vi "SDG60ConfArbWaveform2new.vi"(0 "VISA resource name":refnum<visa-resource-name>="USB0::0xF4EC::0x1101::SDG6XEBC5R0119::INSTR", 1 "DDS/TArb 0: DDS":i32(ring) items=["DDS", "TrueArb"], 2 "Interpolation 0: Zero-order":i32(ring) items=["Zero-Order", "Linear", "Sinc", "Sin27", "Sinc13"], 3 "Offset (0.00 V)":dbl min=-10.0 max=10.0 format="%#_15g", 5 "Select Channel (1:Channel 1)":i32(ring)=1 items=["Channel 1"=1, "Channel 2"=2], 7 "Amplitude(0.1 Vpp)":dbl=0.1 min=0.001 max=20.0 step=1.0 format="%#.15f", 9 "Freq/SR/P (1 Hz)":dbl=1.0 min=1e-06 max=160000000.0 step=1.0 format="%#.15g", 11 "error in (no error)":errorcluster, 12 "Select Freq/SR/P (0:Freq)":i32(ring) items=["Frequency", "Sample Rate", "Period"], 13 "Phase (0 deg)":dbl min=-360.0 max=360.0 format="%#.15g") -> (4 "VISA resource name out":refnum<visa-resource-name>, 15 "error out":errorcluster)   [LabVIEW 2018]
doc: "Sets the waveform parameters for an arbitrary waveform. This VI should be called after <b>Create Arbitrary Waveform.vi</b> (for user defined arbitrary waveform) and <b>Select Arbitrary Waveform.vi</b>"
panel:
  # "Must precede with SDG60SelectArbitraryWFM\nMay take time (~20s) if WFM is large"
  # "Sinc type interpolations use virtual keys\nVirtual keys not used for zero-hold & linear\nInterpolation method, is only for TrueArb\nIf still selected, generator will not make any parameter changes"
  # "Range: 2mVpp-20Vpp. \n6 digits precision"
  # "Range: -10V-10V\n6 digits precision"
  # "Freq (DDS): 1uHz-50MHz \nFreq (TrueArb): 1uHz- Max depends on WFM length\nSR: 1uS/s-300MSa/s\nP: 20ns-1Ms\n10 Digit precision for F & SR\n6 Digit precision for P"
  # "For TrueArb use only F or SR \nFor DDS use F or P\nMay take time (few seconds!) to switch to TrueArb if WFM is large"
  # "Range -360..360deg, larger values will be warped to this range. Resolution 0.0001 deg"
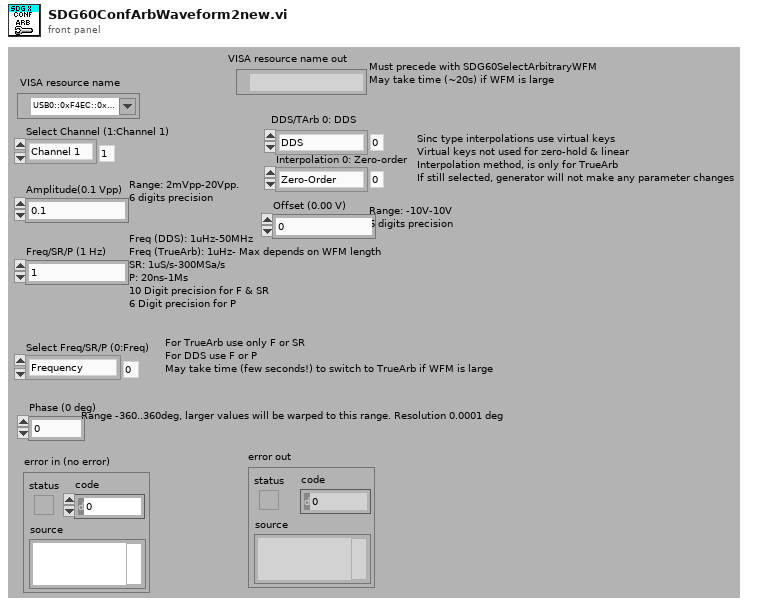
[diagram p1: front panel]
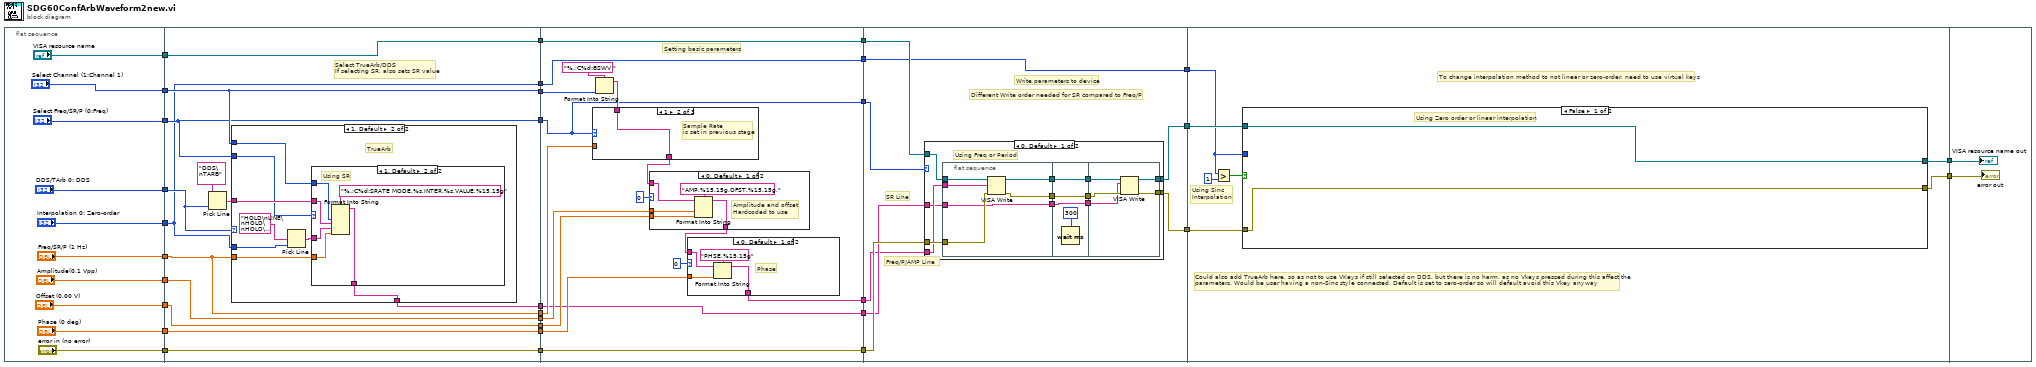
[diagram p0: block diagram]
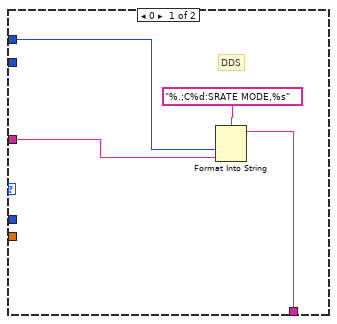
[diagram p2: hidden frame]
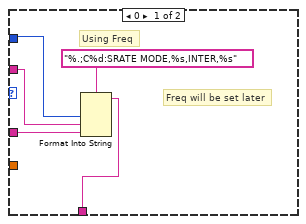
[diagram p3: hidden frame]
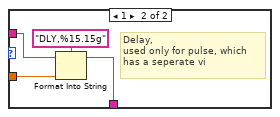
[diagram p4: hidden frame]
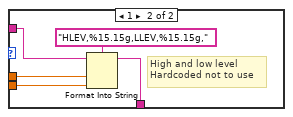
[diagram p5: hidden frame]
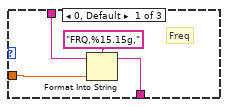
[diagram p6: hidden frame]
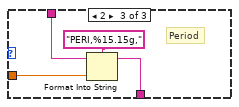
[diagram p7: hidden frame]
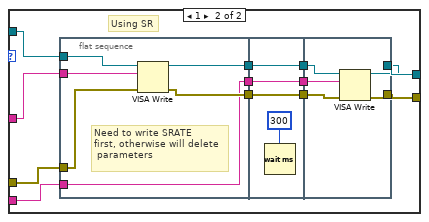
[diagram p8: hidden frame]
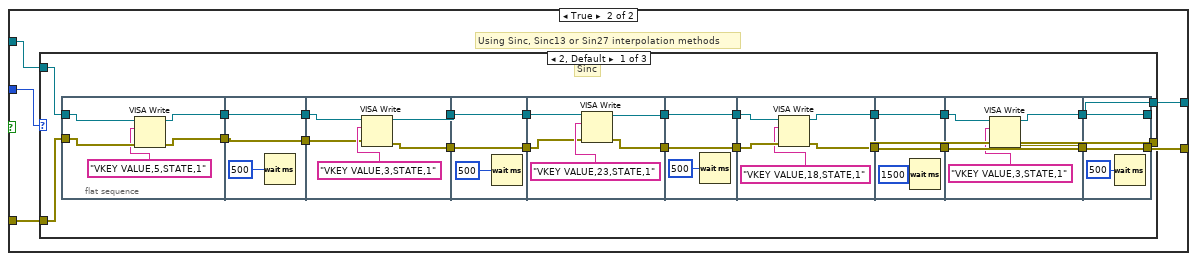
[diagram p9: hidden frame]
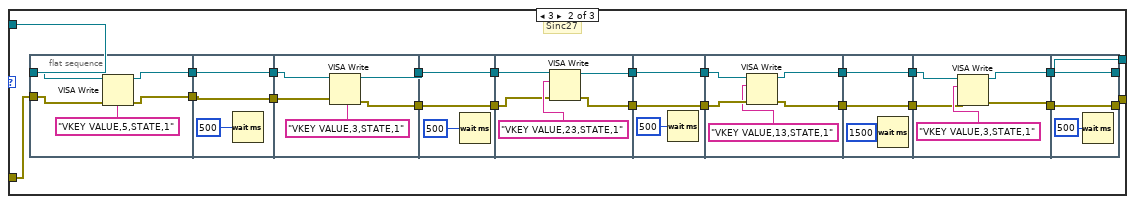
[diagram p10: hidden frame]
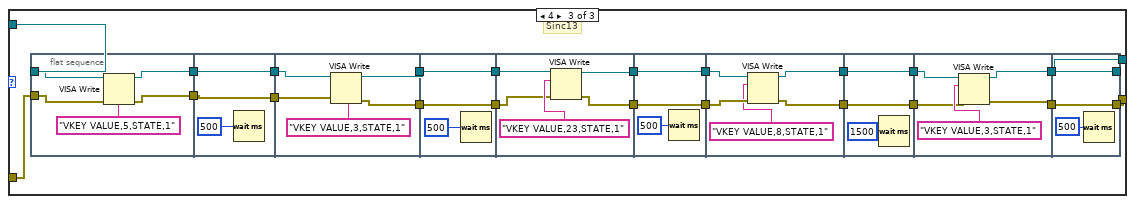
[diagram p11: hidden frame]
diagram:
  n1 = flat-sequence {
    tunnel: ["VISA resource name"] -> w31
    tunnel: ["error in (no error)"] -> w30
    tunnel: ["Amplitude(0.1 Vpp)"] -> w29
    tunnel: ["Phase (0 deg)"] -> w28
    tunnel: ["Freq/SR/P (1 Hz)"] -> w27
    tunnel: ["Offset (0.00 V)"] -> w26
    tunnel: ["Select Freq/SR/P (0:Freq)"] -> w25
    tunnel: ["DDS/TArb 0: DDS"] -> w24
    tunnel: ["Interpolation 0: Zero-order"] -> w23
    tunnel: ["Select Channel (1:Channel 1)"] -> w22
    tunnel: w31 -> [w50]
    tunnel: w30 -> [w54]
    tunnel: w29 -> [w48]
    tunnel: w28 -> [w49]
    tunnel: w27 -> [w47]
    tunnel: w26 -> [w46]
    tunnel: w25 -> [w44]
    tunnel: w24 -> [w51]
    tunnel: w23 -> [w43]
    tunnel: w22 -> [w45]
    tunnel: [w54] -> w21
    tunnel: [w50] -> w19
    tunnel: [w49] -> w17
    tunnel: [w48] -> w16
    tunnel: [w47] -> w15
    tunnel: [w46] -> w14
    tunnel: [w45] -> w13
    tunnel: [w44] -> w12
    tunnel: [w43] -> w11
    tunnel: [w42] -> w9
    tunnel: w21 -> [w94]
    tunnel: [w94] -> w20
    tunnel: w19 -> [w93]
    tunnel: [w93] -> w18
    tunnel: w17 -> [w84]
    tunnel: w16 -> [w86]
    tunnel: w15 -> [w87]
    tunnel: w14 -> [w85]
    tunnel: w13 -> [w88]
    tunnel: w12 -> [w78]
    tunnel: w11 -> [w83]
    tunnel: [w83] -> w10
    tunnel: w9 -> [w82]
    tunnel: [w82] -> w8
    tunnel: [w81] -> w7
    tunnel: [w78] -> w1
    tunnel: w20 -> [w129]
    tunnel: w18 -> [w126]
    tunnel: w10 -> [w123]
    tunnel: w8 -> [w125]
    tunnel: w7 -> [w124]
    tunnel: [w128] -> w6
    tunnel: [w127] -> w5
    tunnel: [w123] -> w4
    tunnel: w1 -> [w122]
    tunnel: w6 -> [w188]
    tunnel: w5 -> [w189]
    tunnel: w4 -> [w184]
    tunnel: [w190] -> w3
    tunnel: [w187] -> w2
    tunnel: w3 -> [w385]
    tunnel: w2 -> [w384]
    frame #0 {
    }
    frame #1 {
      # "Select TrueArb/DDS\nIf selecting SR, also sets SR value"
      n2 = Pick Line(multi-line string="DDS\nTARB", line index=w51) -> (output string=w52:string)  [unwired: 1 in]
      n3 = case shown="1, Default" w51 {
        tunnel: [w57 w66] -> w42
        tunnel: w45 -> [w55 w65]
        tunnel: w52 -> [w56 w64]
        tunnel: w47 -> [_ w61]
        tunnel: w44 -> [_ w60]
        tunnel: w43 -> [_ w59]
        frame 0 {
          # "DDS"
          n4 = Format Into String(format string="%.;C%d:SRATE MODE,%s", w55, w56) -> (resulting string=w57:string)  [unwired: 2 in, 1 out]
        }
        frame 1, Default {
          # "TrueArb"
          n5 = Pick Line(multi-line string="HOLD\nLINE\nHOLD\nHOLD\nHOLD\nHOLD", line index=w59) -> (output string=w62:string)  [unwired: 1 in]
          n6 = case shown="1, Default" w60 {
            tunnel: w65 -> [w70 w76]
            tunnel: [w69 w75] -> w66
            tunnel: w64 -> [w68 w74]
            tunnel: w62 -> [w67 w73]
            tunnel: w61 -> [_ w72]
            frame 0 {
              # "Freq will be set later"
              # "Using Freq"
              n7 = Format Into String(format string="%.;C%d:SRATE MODE,%s,INTER,%s", w70, w68, w67) -> (resulting string=w69:string)  [unwired: 2 in, 1 out]
            }
            frame 1, Default {
              # "Using SR"
              n8 = Format Into String(format string="%.;C%d:SRATE MODE,%s,INTER,%s,VALUE,%15.15g", w76, w74, w73, w72) -> (resulting string=w75:string)  [unwired: 2 in, 1 out]
            }
          }
        }
      }
    }
    frame #2 {
      # "Setting basic parameters"
      n9 = Format Into String(format string="%.;C%d:BSWV ", w88) -> (resulting string=w90:string)  [unwired: 2 in, 1 out]
      n10 = case shown="1" w78 {
        tunnel: w90 -> [w116 w117 w121]
        tunnel: [w114 w117 w119] -> w79
        tunnel: w87 -> [w113 _ w118]
        frame 0, Default {
          # "Freq"
          n11 = Format Into String(format string="FRQ,%15.15g,", initial string=w116, w113) -> (resulting string=w114:string)  [unwired: 1 in, 1 out]
        }
        frame 1 {
          # "Sample Rate\nis set in previous stage"
        }
        frame 2 {
          # "Period"
          n12 = Format Into String(format string="PERI,%15.15g,", initial string=w121, w118) -> (resulting string=w119:string)  [unwired: 1 in, 1 out]
        }
      }
      n13 = case shown="0, Default" 0 {
        tunnel: [w106 w111] -> w80
        tunnel: w86 -> [w105 w110]
        tunnel: w85 -> [w104 w109]
        tunnel: w79 -> [w103 w108]
        frame 0, Default {
          # "Amplitude and offset\nHardcoded to use"
          n14 = Format Into String(format string="AMP,%15.15g,OFST,%15.15g,", initial string=w103, w105, w104) -> (resulting string=w106:string)  [unwired: 1 in, 1 out]
        }
        frame 1 {
          # "High and low level\nHardcoded not to use"
          n15 = Format Into String(format string="HLEV,%15.15g,LLEV,%15.15g,", initial string=w108, w110, w109) -> (resulting string=w111:string)  [unwired: 1 in, 1 out]
        }
      }
      n16 = case shown="0, Default" 0 {
        tunnel: [w97 w101] -> w81
        tunnel: w84 -> [w96 w100]
        tunnel: w80 -> [w95 w99]
        frame 0, Default {
          # "Phase"
          n17 = Format Into String(format string="PHSE,%15.15g", initial string=w95, w96) -> (resulting string=w97:string)  [unwired: 1 in, 1 out]
        }
        frame 1 {
          # "Delay,\nused only for pulse, which \nhas a seperate vi"
          n18 = Format Into String(format string="DLY,%15.15g", initial string=w99, w100) -> (resulting string=w101:string)  [unwired: 1 in, 1 out]
        }
      }
    }
    frame #3 {
      # "Freq/P/AMP Line"
      # "SR Line"
      # "Different Write order needed for SR compared to Freq/P"
      # "Write parameters to device"
      n19 = case shown="0, Default" w122 {
        tunnel: [w137 w164] -> w127
        tunnel: [w136 w163] -> w128
        tunnel: w126 -> [w135 w162]
        tunnel: w129 -> [w134 w161]
        tunnel: w125 -> [w131 w160]
        tunnel: w124 -> [w133 w159]
        frame 0, Default {
          # "Using Freq or Period"
          n20 = flat-sequence {
            tunnel: [w147] -> w141
            tunnel: [w146] -> w140
            tunnel: w135 -> [w145]
            tunnel: w134 -> [w144]
            tunnel: w133 -> [w142]
            tunnel: [w143] -> w132
            tunnel: w131 -> [w143]
            tunnel: w141 -> [w150]
            tunnel: [w150] -> w139
            tunnel: [w149] -> w138
            tunnel: w140 -> [w149]
            tunnel: w132 -> [w148]
            tunnel: [w148] -> w130
            tunnel: [w153] -> w137
            tunnel: w139 -> [w154]
            tunnel: w138 -> [w156]
            tunnel: [w155] -> w136
            tunnel: w130 -> [w152]
            frame #0 {
              n21 = VISA Write(VISA resource name=w145, write buffer=w142, error in (no error)=w144) -> (VISA resource name out=w147:refnum<visa-resource-name>, error out=w146:errorcluster)  [unwired: 1 out]
            }
            frame #1 {
              n22 = Wait (ms)(milliseconds to wait=300 ("x")) -> ()  [unwired: 1 out]
            }
            frame #2 {
              n23 = VISA Write(VISA resource name=w154, write buffer=w152, error in (no error)=w156) -> (VISA resource name out=w153:refnum<visa-resource-name>, error out=w155:errorcluster)  [unwired: 1 out]
            }
          }
        }
        frame 1 {
          # "Using SR"
          n24 = flat-sequence {
            tunnel: [w174] -> w168
            tunnel: [w173] -> w167
            tunnel: w162 -> [w172]
            tunnel: w161 -> [w171]
            tunnel: w160 -> [w169]
            tunnel: w159 -> [w170]
            tunnel: [w170] -> w157
            tunnel: w168 -> [w177]
            tunnel: [w177] -> w166
            tunnel: [w176] -> w165
            tunnel: w167 -> [w176]
            tunnel: [w175] -> w158
            tunnel: w157 -> [w175]
            tunnel: [w180] -> w164
            tunnel: w166 -> [w181]
            tunnel: w165 -> [w183]
            tunnel: [w182] -> w163
            tunnel: w158 -> [w179]
            frame #0 {
              # "Need to write SRATE\nfirst, otherwise will delete\n parameters"
              n25 = VISA Write(VISA resource name=w172, write buffer=w169, error in (no error)=w171) -> (VISA resource name out=w174:refnum<visa-resource-name>, error out=w173:errorcluster)  [unwired: 1 out]
            }
            frame #1 {
              n26 = Wait (ms)(milliseconds to wait=300 ("x")) -> ()  [unwired: 1 out]
            }
            frame #2 {
              n27 = VISA Write(VISA resource name=w181, write buffer=w179, error in (no error)=w183) -> (VISA resource name out=w180:refnum<visa-resource-name>, error out=w182:errorcluster)  [unwired: 1 out]
            }
          }
        }
      }
    }
    frame #4 {
      # "Could also add TrueArb here, so as not to use VKeys if still selected on DDS, but there is no harm, as no Vkeys pressed during this affect the \nparameters. Would be user having a non-Sinc style connected. Default is set to zero-order so will default avoid this Vkey anyway"
      # "Using Sinc \nInterpolation"
      # "To change interpolation method to not linear or zero-order, need to use virtual keys"
      n28 = Greater?(x=w184, y=1) -> (0:w186:bool)
      n29 = case shown="False" w186 {
        tunnel: [w192 w194] -> w190
        tunnel: [w191 w195] -> w187
        tunnel: w189 -> [w192 w197]
        tunnel: w188 -> [w191 w196]
        tunnel: w184 -> [_ w193]
        frame False {
          # "Using Zero order or linear interpolation"
        }
        frame True {
          # "Using Sinc, Sinc13 or Sin27 interpolation methods"
          n30 = case shown="2, Default" w193 {
            tunnel: w197 -> [w214 w276 w338]
            tunnel: w196 -> [w215 w277 w339]
            tunnel: [w212 w274 w336] -> w195
            tunnel: [w213 w275 w337] -> w194
            frame 2, Default {
              # "Sinc"
              n31 = flat-sequence {
                tunnel: w215 -> [w224]
                tunnel: w214 -> [w223]
                tunnel: [w222] -> w219
                tunnel: [w220] -> w218
                tunnel: w219 -> [w227]
                tunnel: [w227] -> w217
                tunnel: [w225] -> w216
                tunnel: w218 -> [w225]
                tunnel: w217 -> [w231]
                tunnel: w216 -> [w228]
                tunnel: [w230] -> w211
                tunnel: [w229] -> w210
                tunnel: w211 -> [w235]
                tunnel: [w235] -> w209
                tunnel: w210 -> [w234]
                tunnel: [w234] -> w207
                tunnel: w209 -> [w240]
                tunnel: [w236] -> w208
                tunnel: w207 -> [w238]
                tunnel: [w237] -> w206
                tunnel: w208 -> [w243]
                tunnel: w206 -> [w242]
                tunnel: [w243] -> w205
                tunnel: [w242] -> w204
                tunnel: w205 -> [w248]
                tunnel: w204 -> [w247]
                tunnel: [w245] -> w203
                tunnel: [w246] -> w202
                tunnel: w203 -> [w251]
                tunnel: w202 -> [w250]
                tunnel: [w251] -> w201
                tunnel: [w250] -> w200
                tunnel: w201 -> [w256]
                tunnel: w200 -> [w253]
                tunnel: [w255] -> w199
                tunnel: [w252] -> w198
                tunnel: [w258] -> w212
                tunnel: [w259] -> w213
                tunnel: w199 -> [w259]
                tunnel: w198 -> [w258]
                frame #0 {
                  n32 = VISA Write(VISA resource name=w223, write buffer="VKEY VALUE,5,STATE,1", error in (no error)=w224) -> (VISA resource name out=w222:refnum<visa-resource-name>, error out=w220:errorcluster)  [unwired: 1 out]
                }
                frame #1 {
                  n33 = Wait (ms)(milliseconds to wait=500) -> ()  [unwired: 1 out]
                }
                frame #2 {
                  n34 = VISA Write(VISA resource name=w231, write buffer="VKEY VALUE,3,STATE,1", error in (no error)=w228) -> (VISA resource name out=w230:refnum<visa-resource-name>, error out=w229:errorcluster)  [unwired: 1 out]
                }
                frame #3 {
                  n35 = Wait (ms)(milliseconds to wait=500) -> ()  [unwired: 1 out]
                }
                frame #4 {
                  n36 = VISA Write(VISA resource name=w240, write buffer="VKEY VALUE,23,STATE,1", error in (no error)=w238) -> (VISA resource name out=w236:refnum<visa-resource-name>, error out=w237:errorcluster)  [unwired: 1 out]
                }
                frame #5 {
                  n37 = Wait (ms)(milliseconds to wait=500) -> ()  [unwired: 1 out]
                }
                frame #6 {
                  n38 = VISA Write(VISA resource name=w248, write buffer="VKEY VALUE,18,STATE,1", error in (no error)=w247) -> (VISA resource name out=w245:refnum<visa-resource-name>, error out=w246:errorcluster)  [unwired: 1 out]
                }
                frame #7 {
                  n39 = Wait (ms)(milliseconds to wait=1500) -> ()  [unwired: 1 out]
                }
                frame #8 {
                  n40 = VISA Write(VISA resource name=w256, write buffer="VKEY VALUE,3,STATE,1", error in (no error)=w253) -> (VISA resource name out=w255:refnum<visa-resource-name>, error out=w252:errorcluster)  [unwired: 1 out]
                }
                frame #9 {
                  n41 = Wait (ms)(milliseconds to wait=500) -> ()  [unwired: 1 out]
                }
              }
            }
            frame 3 {
              # "Sinc27"
              n42 = flat-sequence {
                tunnel: w277 -> [w286]
                tunnel: w276 -> [w285]
                tunnel: [w284] -> w281
                tunnel: [w282] -> w280
                tunnel: w281 -> [w289]
                tunnel: [w289] -> w279
                tunnel: [w287] -> w278
                tunnel: w280 -> [w287]
                tunnel: w279 -> [w293]
                tunnel: w278 -> [w290]
                tunnel: [w292] -> w273
                tunnel: [w291] -> w272
                tunnel: w273 -> [w297]
                tunnel: [w297] -> w271
                tunnel: w272 -> [w296]
                tunnel: [w296] -> w269
                tunnel: w271 -> [w302]
                tunnel: [w298] -> w270
                tunnel: w269 -> [w300]
                tunnel: [w299] -> w268
                tunnel: w270 -> [w305]
                tunnel: w268 -> [w304]
                tunnel: [w305] -> w267
                tunnel: [w304] -> w266
                tunnel: w267 -> [w310]
                tunnel: w266 -> [w309]
                tunnel: [w307] -> w265
                tunnel: [w308] -> w264
                tunnel: w265 -> [w313]
                tunnel: w264 -> [w312]
                tunnel: [w313] -> w263
                tunnel: [w312] -> w262
                tunnel: w263 -> [w318]
                tunnel: w262 -> [w315]
                tunnel: [w317] -> w261
                tunnel: [w314] -> w260
                tunnel: [w320] -> w274
                tunnel: [w321] -> w275
                tunnel: w261 -> [w321]
                tunnel: w260 -> [w320]
                frame #0 {
                  n43 = VISA Write(VISA resource name=w285, write buffer="VKEY VALUE,5,STATE,1", error in (no error)=w286) -> (VISA resource name out=w284:refnum<visa-resource-name>, error out=w282:errorcluster)  [unwired: 1 out]
                }
                frame #1 {
                  n44 = Wait (ms)(milliseconds to wait=500) -> ()  [unwired: 1 out]
                }
                frame #2 {
                  n45 = VISA Write(VISA resource name=w293, write buffer="VKEY VALUE,3,STATE,1", error in (no error)=w290) -> (VISA resource name out=w292:refnum<visa-resource-name>, error out=w291:errorcluster)  [unwired: 1 out]
                }
                frame #3 {
                  n46 = Wait (ms)(milliseconds to wait=500) -> ()  [unwired: 1 out]
                }
                frame #4 {
                  n47 = VISA Write(VISA resource name=w302, write buffer="VKEY VALUE,23,STATE,1", error in (no error)=w300) -> (VISA resource name out=w298:refnum<visa-resource-name>, error out=w299:errorcluster)  [unwired: 1 out]
                }
                frame #5 {
                  n48 = Wait (ms)(milliseconds to wait=500) -> ()  [unwired: 1 out]
                }
                frame #6 {
                  n49 = VISA Write(VISA resource name=w310, write buffer="VKEY VALUE,13,STATE,1", error in (no error)=w309) -> (VISA resource name out=w307:refnum<visa-resource-name>, error out=w308:errorcluster)  [unwired: 1 out]
                }
                frame #7 {
                  n50 = Wait (ms)(milliseconds to wait=1500) -> ()  [unwired: 1 out]
                }
                frame #8 {
                  n51 = VISA Write(VISA resource name=w318, write buffer="VKEY VALUE,3,STATE,1", error in (no error)=w315) -> (VISA resource name out=w317:refnum<visa-resource-name>, error out=w314:errorcluster)  [unwired: 1 out]
                }
                frame #9 {
                  n52 = Wait (ms)(milliseconds to wait=500) -> ()  [unwired: 1 out]
                }
              }
            }
            frame 4 {
              # "Sinc13"
              n53 = flat-sequence {
                tunnel: w339 -> [w348]
                tunnel: w338 -> [w347]
                tunnel: [w346] -> w343
                tunnel: [w344] -> w342
                tunnel: w343 -> [w351]
                tunnel: [w351] -> w341
                tunnel: [w349] -> w340
                tunnel: w342 -> [w349]
                tunnel: w341 -> [w355]
                tunnel: w340 -> [w352]
                tunnel: [w354] -> w335
                tunnel: [w353] -> w334
                tunnel: w335 -> [w359]
                tunnel: [w359] -> w333
                tunnel: w334 -> [w358]
                tunnel: [w358] -> w331
                tunnel: w333 -> [w364]
                tunnel: [w360] -> w332
                tunnel: w331 -> [w362]
                tunnel: [w361] -> w330
                tunnel: w332 -> [w367]
                tunnel: w330 -> [w366]
                tunnel: [w367] -> w329
                tunnel: [w366] -> w328
                tunnel: w329 -> [w372]
                tunnel: w328 -> [w371]
                tunnel: [w369] -> w327
                tunnel: [w370] -> w326
                tunnel: w327 -> [w375]
                tunnel: w326 -> [w374]
                tunnel: [w375] -> w325
                tunnel: [w374] -> w324
                tunnel: w325 -> [w380]
                tunnel: w324 -> [w377]
                tunnel: [w379] -> w323
                tunnel: [w376] -> w322
                tunnel: [w382] -> w336
                tunnel: [w383] -> w337
                tunnel: w323 -> [w383]
                tunnel: w322 -> [w382]
                frame #0 {
                  n54 = VISA Write(VISA resource name=w347, write buffer="VKEY VALUE,5,STATE,1", error in (no error)=w348) -> (VISA resource name out=w346:refnum<visa-resource-name>, error out=w344:errorcluster)  [unwired: 1 out]
                }
                frame #1 {
                  n55 = Wait (ms)(milliseconds to wait=500) -> ()  [unwired: 1 out]
                }
                frame #2 {
                  n56 = VISA Write(VISA resource name=w355, write buffer="VKEY VALUE,3,STATE,1", error in (no error)=w352) -> (VISA resource name out=w354:refnum<visa-resource-name>, error out=w353:errorcluster)  [unwired: 1 out]
                }
                frame #3 {
                  n57 = Wait (ms)(milliseconds to wait=500) -> ()  [unwired: 1 out]
                }
                frame #4 {
                  n58 = VISA Write(VISA resource name=w364, write buffer="VKEY VALUE,23,STATE,1", error in (no error)=w362) -> (VISA resource name out=w360:refnum<visa-resource-name>, error out=w361:errorcluster)  [unwired: 1 out]
                }
                frame #5 {
                  n59 = Wait (ms)(milliseconds to wait=500) -> ()  [unwired: 1 out]
                }
                frame #6 {
                  n60 = VISA Write(VISA resource name=w372, write buffer="VKEY VALUE,8,STATE,1", error in (no error)=w371) -> (VISA resource name out=w369:refnum<visa-resource-name>, error out=w370:errorcluster)  [unwired: 1 out]
                }
                frame #7 {
                  n61 = Wait (ms)(milliseconds to wait=1500) -> ()  [unwired: 1 out]
                }
                frame #8 {
                  n62 = VISA Write(VISA resource name=w380, write buffer="VKEY VALUE,3,STATE,1", error in (no error)=w377) -> (VISA resource name out=w379:refnum<visa-resource-name>, error out=w376:errorcluster)  [unwired: 1 out]
                }
                frame #9 {
                  n63 = Wait (ms)(milliseconds to wait=500) -> ()  [unwired: 1 out]
                }
              }
            }
          }
        }
      }
    }
    frame #5 {
      "VISA resource name out" <- w385
      "error out" <- w384
    }
  }
